vi "Remove_Duplicate_QDC_Data.vi"(1 "Input Data":T2(array[cluster])) -> (0 "Output Data":T1(array[cluster]))   [LabVIEW 2014]
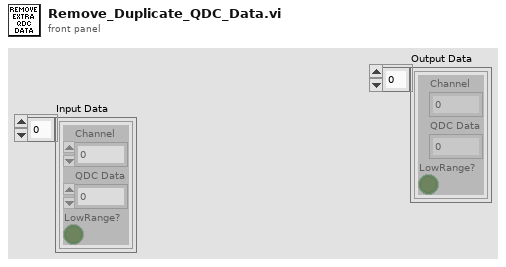
[diagram p1: front panel]
types:
  T1 = cluster{"Channel":u8, "QDC Data":u16, "LowRange?":bool}[]
  T2 = cluster{"Channel":u8, "QDC Data":sgl, "LowRange?":bool}[]
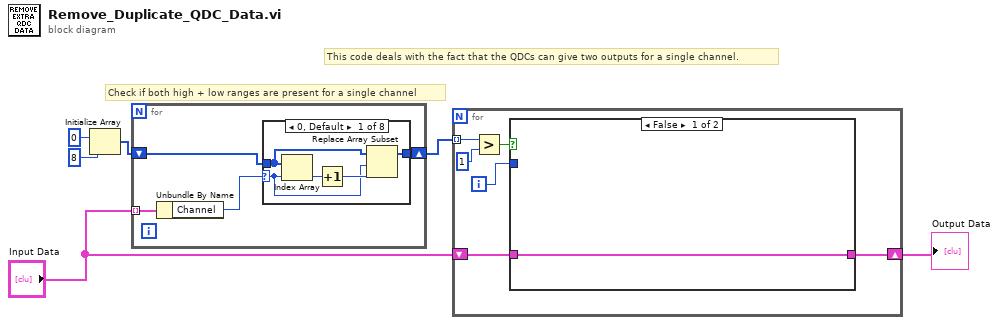
[diagram p0: block diagram]
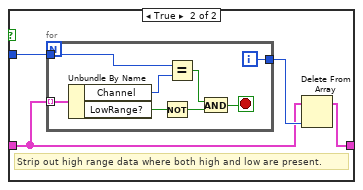
[diagram p2: hidden frame]
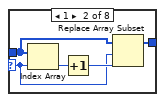
[diagram p3: hidden frame]
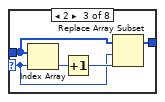
[diagram p4: hidden frame]
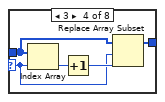
[diagram p5: hidden frame]
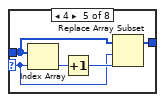
[diagram p6: hidden frame]
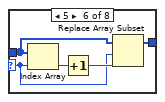
[diagram p7: hidden frame]
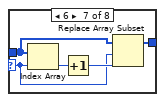
[diagram p8: hidden frame]
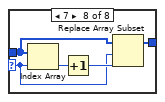
[diagram p9: hidden frame]
diagram:
  # "This code deals with the fact that the QDCs can give two outputs for a single channel."
  # "Check if both high + low ranges are present for a single channel"
  n1 = Initialize Array(u16 0 ("element"), 8 ("dimension size")) -> (w4:u16[])
  n2 = for {
    tunnel: "Input Data" -> [w10] mode=indexing
    shift-right: [w7] -> w3
    shift-left: w4 -> [w8]
    n3 = Unbundle By Name(w10) -> ("Channel"=w9:u8)
    n4 = case shown="0, Default" w9 {
      selector: w9 -> [w12 w17 w22 w27 w32 w37 w42 w47]
      tunnel: w8 -> [w13 w18 w23 w28 w33 w38 w43 w48]
      tunnel: [w11 w16 w21 w26 w31 w36 w41 w46] -> w7
      frame 0, Default {
        n5 = Index Array(array=w13, index=w12) -> (element=w15:u16)
        n6 = Increment(x=w15) -> (x+1=w14:u16)
        n7 = Replace Array Subset(array=w13, new element=w14, index=w12) -> (w11:u16[])
      }
      frame 1 {
        n8 = Index Array(array=w18, index=w17) -> (element=w20:u16)
        n9 = Increment(x=w20) -> (x+1=w19:u16)
        n10 = Replace Array Subset(array=w18, new element=w19, index=w17) -> (w16:u16[])
      }
      frame 2 {
        n11 = Index Array(array=w23, index=w22) -> (element=w25:u16)
        n12 = Increment(x=w25) -> (x+1=w24:u16)
        n13 = Replace Array Subset(array=w23, new element=w24, index=w22) -> (w21:u16[])
      }
      frame 3 {
        n14 = Index Array(array=w28, index=w27) -> (element=w30:u16)
        n15 = Increment(x=w30) -> (x+1=w29:u16)
        n16 = Replace Array Subset(array=w28, new element=w29, index=w27) -> (w26:u16[])
      }
      frame 4 {
        n17 = Index Array(array=w33, index=w32) -> (element=w35:u16)
        n18 = Increment(x=w35) -> (x+1=w34:u16)
        n19 = Replace Array Subset(array=w33, new element=w34, index=w32) -> (w31:u16[])
      }
      frame 5 {
        n20 = Index Array(array=w38, index=w37) -> (element=w40:u16)
        n21 = Increment(x=w40) -> (x+1=w39:u16)
        n22 = Replace Array Subset(array=w38, new element=w39, index=w37) -> (w36:u16[])
      }
      frame 6 {
        n23 = Index Array(array=w43, index=w42) -> (element=w45:u16)
        n24 = Increment(x=w45) -> (x+1=w44:u16)
        n25 = Replace Array Subset(array=w43, new element=w44, index=w42) -> (w41:u16[])
      }
      frame 7 {
        n26 = Index Array(array=w48, index=w47) -> (element=w50:u16)
        n27 = Increment(x=w50) -> (x+1=w49:u16)
        n28 = Replace Array Subset(array=w48, new element=w49, index=w47) -> (w46:u16[])
      }
    }
  }
  n29 = for {
    tunnel: w3 -> [w56] mode=indexing
    shift-right: [w51] -> w1
    shift-left: "Input Data" -> [w52]
    i -> [w53]
    n30 = Greater?(x=w56, y=u8 1) -> (0:w54:bool)
    n31 = case shown="False" w54 {
      tunnel: w53 -> [_ w61]
      tunnel: w52 -> [w57 w59]
      tunnel: [w57 w58] -> w51
      frame False {
      }
      frame True {
        # "Strip out high range data where both high and low are present."
        n32 = for {
          tunnel: w59 -> [w69] mode=indexing
          tunnel: w61 -> [w65]
          tunnel: [w68] -> w60
          i -> [w68]
          stop <- w62 stop-if-true
          n33 = Unbundle By Name(w69) -> ("Channel"=w64:u8, "LowRange?"=w67:bool)
          n34 = Not(x=w67) -> (.not. x?=w66:bool)
          n35 = Equal?(x=w65, y=w64) -> (x = y?=w63:bool)
          n36 = And(x=w63, y=w66) -> (x .and. y?=w62:bool)
        }
        n37 = Delete From Array(array=w59, index=w60) -> (array with subset deleted=w58:T2)  [unwired: 1 in, 1 out]
      }
    }
  }
  "Output Data" <- w1
